vi "Test_9.vi"(11 "bool_in":bool) -> (3 "bool_out":bool)   [LabVIEW 2020]
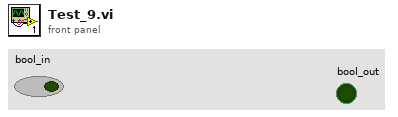
[diagram p1: front panel]
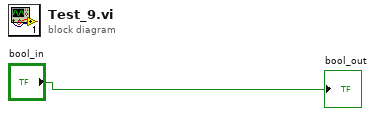
[diagram p0: block diagram]
diagram:
  "bool_out" <- "bool_in"
